vi "Set PID.vi"(8 "error in (no error)":errorcluster, 10 "PID":T1, 11 "SimPID in":refnum<class "SimPID.lvclass">) -> (0 "error out":errorcluster, 3 "SimPID out":refnum<class "SimPID.lvclass">)   [LabVIEW 2023, in "SimPID.lvclass"]
uses:
  SimPID.lvclass
  SimPID.lvclass/SimPID.ctl
  PIDController/PIDController.lvclass
  PIDModBus/Controls/PID Cluster.ctl
  PIDModBus/PIDModbus.lvlib
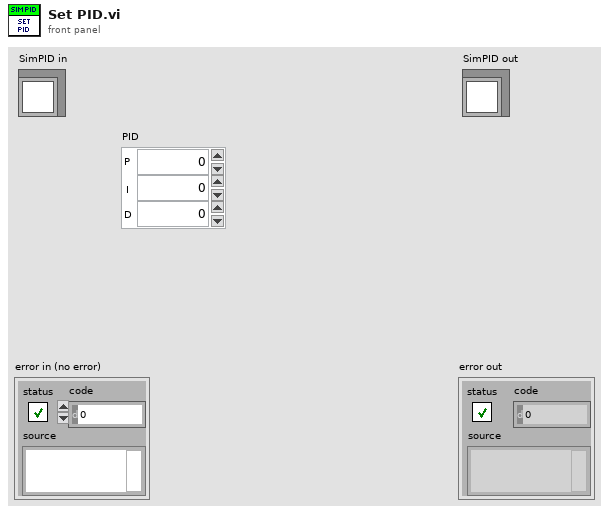
[diagram p1: front panel]
types:
  T1 = typedef "PIDModbus.lvlib/PID Cluster.ctl" = cluster{"P":u16, "I":u16, "D":u16}
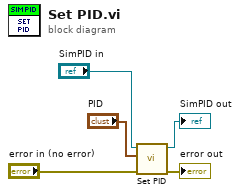
[diagram p0: block diagram]
diagram:
  n1 = call-parent "Set PID.vi"("error in (no error)"="error in (no error)", "PID"="PID", "PIDController in"="SimPID in") -> ("error out"=→"error out":errorcluster, "PIDController out"=→"SimPID out":refnum<class "SimPID.lvclass">)  [unwired: 7 in]
